vi "ReceiveFIFO_FromFPGA.vi"(7 "Num Samples":u32, 8 "error in (no error)":errorcluster, 9 "queue in":refnum<queue>, 10 "SampleRate":dbl=12500.0, 11 "FPGA Ref in":refnum<k20>) -> (0 "error out":errorcluster, 2 "Elements Remaining":u32, 3 "Refnum out":refnum<k20>)   [LabVIEW 2018]
uses:
  <vilib>/Utility/error.llb/Error Cluster From Error Code.vi
  <vilib>/rvi/errors/niLvFpgaAdjustHostInterfaceError.vi
  <vilib>/rvi/interface/nirviMethod/nirviMethod.xnode
  <vilib>/FPGAPlugInAG/Dynamic/niLvFpga_ReadFifo_Dynamic.vi
  <vilib>/rvi/errors/niLvFpgaMergeErrorWithErrorCode.vi
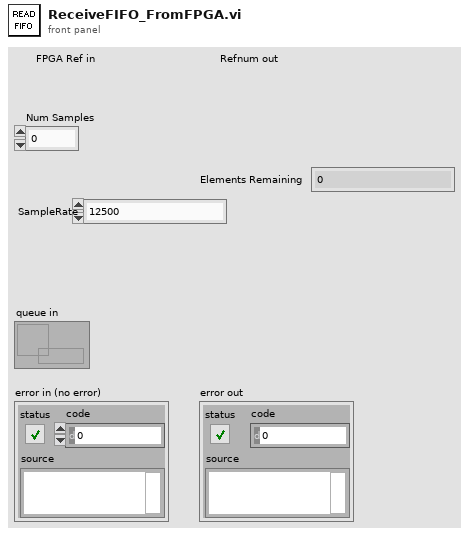
[diagram p1: front panel]
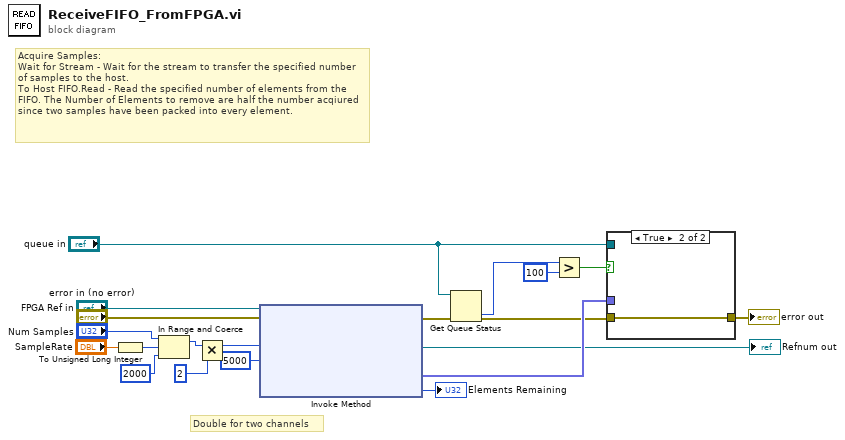
[diagram p0: block diagram]
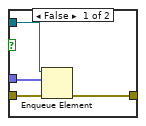
[diagram p2: hidden frame]
diagram:
  # "Double for two channels"
  # "Acquire Samples:\nWait for Stream - Wait for the stream to transfer the specified number of samples to the host.\nTo Host FIFO.Read - Read the specified number of elements from the FIFO. The Number of Elements to remove are half the number acqiured since two samples have been packed into every element."
  n1 = To Unsigned Long Integer(number="SampleRate") -> (unsigned 32bit integer=w17:u32)
  n2 = In Range and Coerce(upper limit="Num Samples", x=w17, lower limit=u32 2000) -> (coerced(x)=w15:u32)  [unwired: 1 out]
  n3 = Multiply(x=w15, y=u32 2) -> (x*y=w18:u32)
  n4 = xnode "Invoke Method"("FPGA VI Reference In"="FPGA Ref in", "error in"="error in (no error)", "Number of Elements"=w18, "Timeout (ms)"=5000) -> ("FPGA VI Reference Out"=→"Refnum out":refnum<k20>, "error out"=w5:errorcluster, "Data"=w13:fxp<+/-,40,1>[], "Elements Remaining"=→"Elements Remaining":u32)
  n5 = Get Queue Status(queue="queue in", error in (no error)=w5) -> (error out=w6:errorcluster, # elements in queue=w3:i32)  [unwired: 1 in, 6 out]
  n6 = Greater?(x=w3, y=100) -> (0:w7:bool)
  n7 = case shown="True" w7 {
    tunnel: w13 -> [w24 _]
    tunnel: "queue in" -> [w23 _]
    tunnel: w6 -> [w22 w25]
    tunnel: [w21 w25] -> w20
    frame False {
      n8 = Enqueue Element(queue=w23, element=w24, error in (no error)=w22) -> (error out=w21:errorcluster)  [unwired: 1 in, 2 out]
    }
    frame True {
    }
  }
  "error out" <- w20
